vi "Arrays Equal (DBL).vi"(1 "Array 2":dbl[](array[numeric]), 2 "Array 1":dbl[](array[numeric])) -> (0 "arrays equal?":bool)   [LabVIEW 2020]
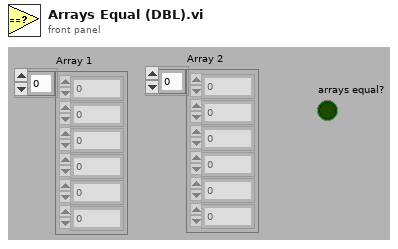
[diagram p1: front panel]
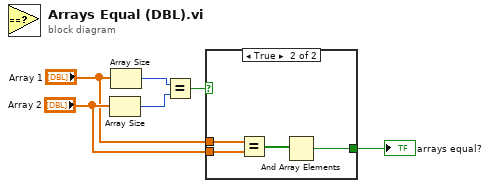
[diagram p0: block diagram]
diagram:
  n1 = Array Size(array="Array 2") -> (size(s)=w5:i32)
  n2 = Array Size(array="Array 1") -> (size(s)=w6:i32)
  n3 = Equal?(x=w6, y=w5) -> (x = y?=w4:bool)
  n4 = case shown="True" w4 {
    selector: w4 -> [w7 _]
    tunnel: [w7 w8] -> w3
    tunnel: "Array 2" -> [_ w11]
    tunnel: "Array 1" -> [_ w10]
    frame False {
    }
    frame True {
      n5 = Equal?(x=w10, y=w11) -> (x = y?=w9:bool[])
      n6 = And Array Elements(Boolean array=w9) -> (logical AND=w8:bool)
    }
  }
  "arrays equal?" <- w3
